vi "MGCC_FntStaMach_Reset.vi"(10 "Input State":string[](array[string])) -> (2 "Output State":string[](array[string]))   [LabVIEW 2016]
uses:
  MGCC_FntStaMach_gobal.vi
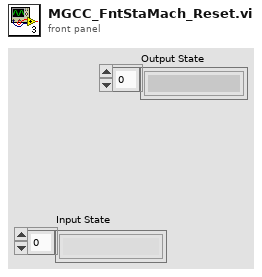
[diagram p1: front panel]
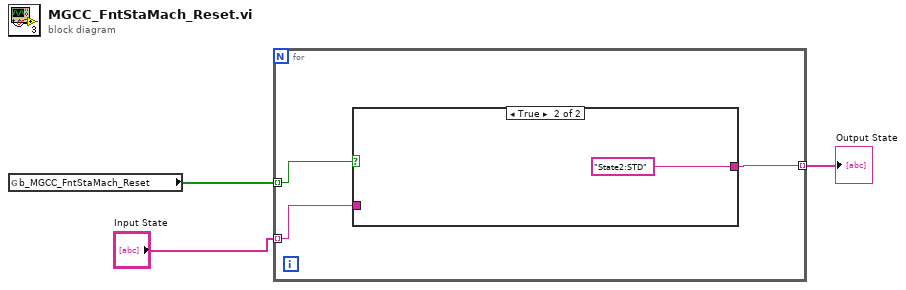
[diagram p0: block diagram]
diagram:
  n1 = global read "MGCC_FntStaMach_gobal.vi" "b_MGCC_FntStaMach_Reset"() -> (w3:bool[])
  n2 = for {
    tunnel: w3 -> [w6] mode=indexing
    tunnel: [w5] -> w1 mode=indexing
    tunnel: "Input State" -> [w4] mode=indexing
    n3 = case shown="True" w6 {
      tunnel: [w7 "State2:STD"] -> w5
      tunnel: w4 -> [w7 _]
      frame False {
      }
      frame True {
      }
    }
  }
  "Output State" <- w1
